vi "WriteToTarget_20190401.vi"(8 "error in":errorcluster, 11 "Tones":T1={"Config"={"UsrCfg"={"Paths"={"CfgFile"=path "", "LogFolder"=path "", "LogFile"=path "", "NAS path"=path "", "ThreshFile"=path "", "RedunFolder"=path ""}, "SampleRate"=0.0}, "FP_User"={"#NoiseSums"=1, "Max_df"=1, "AvgAvg"=FALSE, "#Avg"=0, "AutoCenter"=FALSE, "Inclin"={"Vmin"=0.0, "Vmax"=0.0, "Angle_min"=0.0, "Angle_max"=0.0, "Offset"=0.0, "Pos_Neg"=FALSE}, "1"={"Cal_"={"Fine"=0.0, "Coarse_"=0.0}, "Beac"={"Fine"=0.0, "Coarse_"=0.0}, "Scale"={"Step4"=0.0, "Step5"=0.0, "Step6"=0.0, "Step7"=0.0}, "Offset"=0.0, "Scale_Noise"=0.0, "Scale_Step1"=0.0, "Scale_In_RT"=0.0, "ScaleMeas"=0.0, "FreqsToRemove"=[], "Width"=[0, 1633], "ScaleMeasEnum"=enum."50", "FilterEnab"=enum."Step 1"}, "2"={"Cal_"={"Fine"=0.0, "Coarse_"=0.0}, "Beac"={"Fine"=0.0, "Coarse_"=0.0}, "Scale"={"Step4"=0.0, "Step5"=0.0, "Step6"=0.0, "Step7"=0.0}, "Offset"=0.0, "Scale_Noise"=0.0, "Scale_Step1"=0.0, "Scale_In_RT"=0.0, "ScaleMeas"=0.0, "FreqsToRemove"=[], "Width"=[0, 1633], "ScaleMeasEnum"=enum."50", "FilterEnab"=enum."Step 1"}, "3"={"Cal_"={"Fine"=0.0, "Coarse_"=0.0}, "Beac"={"Fine"=0.0, "Coarse_"=0.0}, "Scale"={"Step4"=0.0, "Step5"=0.0, "Step6"=0.0, "Step7"=0.0}, "Offset"=0.0, "Scale_Noise"=0.0, "Scale_Step1"=0.0, "Scale_In_RT"=0.0, "ScaleMeas"=0.0, "FreqsToRemove"=[], "Width"=[0, 1633], "ScaleMeasEnum"=enum."50", "FilterEnab"=enum."Step 1"}, "4"={"Cal_"={"Fine"=0.0, "Coarse_"=0.0}, "Beac"={"Fine"=0.0, "Coarse_"=0.0}, "Scale"={"Step4"=0.0, "Step5"=0.0, "Step6"=0.0, "Step7"=0.0}, "Offset"=0.0, "Scale_Noise"=0.0, "Scale_Step1"=0.0, "Scale_In_RT"=0.0, "ScaleMeas"=0.0, "FreqsToRemove"=[], "Width"=[0, 1633], "ScaleMeasEnum"=enum."50", "FilterEnab"=enum."Step 1"}, "Target to Probe"=enum."4", "SNR_Thresh"=1.0, "Paths"={"CfgFile"=path "", "LogFolder"=path "", "LogFile"=path "", "NAS path"=path "", "ThreshFile"=path "", "RedunFolder"=path ""}, "Connex_Location"="", "SimulateFPGA"=FALSE, "Deadband"=0.0}}, "FPGA"={"Target"=enum."4", "Channel"=enum."4", "Ref1"=refnum, "Ref2"=refnum}, "Now"={"Target"=enum."1", "SampleRate"=0.0, "AvgFreq"=0.0, "72_Shift_"=-24999462.633451957, "84_Shift_"=-24999462.633451957, "1"={"Cal"={"Shift_"=0.0, "Peak_ToFPGA"=-24999462.633451957, "MaxValue"=0.0, "MaxIndex"=0, "Tone"={"PkLocTrak"=0.0, "PkLocDisp"=0.0, "df_"=0.0, "ZoomPwr"=[], "Phase"=0.0, "PhaseOld"=0.0, "AboveThresh?"=FALSE, "MaxI"=0.0, "MaxQ"=0.0, "median"=0.0, "ISpect"=[], "QSpect"=[], "DeltaPhase"=0.0}, "TimeDomainI"=[], "TimeDomainQ"=array[12500 elements], "PwrSpectrum"=[], "RunningAvgFreq"=0.0, "ISpectPos"=[], "ISpectNeg"=[], "QSpectPos"=[], "QSpectNeg"=[], "10Hz_PwrSpectr"=[], "SNR"=0.0, "AliasWarn"=FALSE, "10Hz_Peak"=[], "ISpect+-"=[], "QSpect+-"=[], "TimeStamp"=timestamp(0 s since 1904-01-01), "I_Index"=array[12500 elements], "Q_Index"=array[12500 elements], "10MHz"=FALSE}, "Beac"={"Shift_"=0.0, "Peak_ToFPGA"=-24999462.633451957, "MaxValue"=0.0, "MaxIndex"=0, "Tone"={"PkLocTrak"=0.0, "PkLocDisp"=0.0, "df_"=0.0, "ZoomPwr"=[], "Phase"=0.0, "PhaseOld"=0.0, "AboveThresh?"=FALSE, "MaxI"=0.0, "MaxQ"=0.0, "median"=0.0, "ISpect"=[], "QSpect"=[], "DeltaPhase"=0.0}, "TimeDomainI"=[], "TimeDomainQ"=array[12500 elements], "PwrSpectrum"=[], "RunningAvgFreq"=0.0, "ISpectPos"=[], "ISpectNeg"=[], "QSpectPos"=[], "QSpectNeg"=[], "10Hz_PwrSpectr"=[], "SNR"=0.0, "AliasWarn"=FALSE, "10Hz_Peak"=[], "ISpect+-"=[], "QSpect+-"=[], "TimeStamp"=timestamp(0 s since 1904-01-01), "I_Index"=array[12500 elements], "Q_Index"=array[12500 elements], "10MHz"=FALSE}, "Time"=[], "Saturat"={"MeasMean0"=0.0, "MeasMean1"=0.0, "MeasMax"=0.0, "1_Max"=0.0, "4_Max"=0.0, "5_Max"=0.0, "6_Max"=0.0, "7_Max"=0.0}}, "2"={"Cal"={"Shift_"=0.0, "Peak_ToFPGA"=-24999462.633451957, "MaxValue"=0.0, "MaxIndex"=0, "Tone"={"PkLocTrak"=0.0, "PkLocDisp"=0.0, "df_"=0.0, "ZoomPwr"=[], "Phase"=0.0, "PhaseOld"=0.0, "AboveThresh?"=FALSE, "MaxI"=0.0, "MaxQ"=0.0, "median"=0.0, "ISpect"=[], "QSpect"=[], "DeltaPhase"=0.0}, "TimeDomainI"=[], "TimeDomainQ"=array[12500 elements], "PwrSpectrum"=[], "RunningAvgFreq"=0.0, "ISpectPos"=[], "ISpectNeg"=[], "QSpectPos"=[], "QSpectNeg"=[], "10Hz_PwrSpectr"=[], "SNR"=0.0, "AliasWarn"=FALSE, "10Hz_Peak"=[], "ISpect+-"=[], "QSpect+-"=[], "TimeStamp"=timestamp(0 s since 1904-01-01), "I_Index"=array[12500 elements], "Q_Index"=array[12500 elements], "10MHz"=FALSE}, "Beac"={"Shift_"=0.0, "Peak_ToFPGA"=-24999462.633451957, "MaxValue"=0.0, "MaxIndex"=0, "Tone"={"PkLocTrak"=0.0, "PkLocDisp"=0.0, "df_"=0.0, "ZoomPwr"=[], "Phase"=0.0, "PhaseOld"=0.0, "AboveThresh?"=FALSE, "MaxI"=0.0, "MaxQ"=0.0, "median"=0.0, "ISpect"=[], "QSpect"=[], "DeltaPhase"=0.0}, "TimeDomainI"=[], "TimeDomainQ"=array[12500 elements], "PwrSpectrum"=[], "RunningAvgFreq"=0.0, "ISpectPos"=[], "ISpectNeg"=[], "QSpectPos"=[], "QSpectNeg"=[], "10Hz_PwrSpectr"=[], "SNR"=0.0, "AliasWarn"=FALSE, "10Hz_Peak"=[], "ISpect+-"=[], "QSpect+-"=[], "TimeStamp"=timestamp(0 s since 1904-01-01), "I_Index"=array[12500 elements], "Q_Index"=array[12500 elements], "10MHz"=FALSE}, "Time"=[], "Saturat"={"MeasMean0"=0.0, "MeasMean1"=0.0, "MeasMax"=0.0, "1_Max"=0.0, "4_Max"=0.0, "5_Max"=0.0, "6_Max"=0.0, "7_Max"=0.0}}, "3"={"Cal"={"Shift_"=0.0, "Peak_ToFPGA"=-24999462.633451957, "MaxValue"=0.0, "MaxIndex"=0, "Tone"={"PkLocTrak"=0.0, "PkLocDisp"=0.0, "df_"=0.0, "ZoomPwr"=[], "Phase"=0.0, "PhaseOld"=0.0, "AboveThresh?"=FALSE, "MaxI"=0.0, "MaxQ"=0.0, "median"=0.0, "ISpect"=[], "QSpect"=[], "DeltaPhase"=0.0}, "TimeDomainI"=[], "TimeDomainQ"=array[12500 elements], "PwrSpectrum"=[], "RunningAvgFreq"=0.0, "ISpectPos"=[], "ISpectNeg"=[], "QSpectPos"=[], "QSpectNeg"=[], "10Hz_PwrSpectr"=[], "SNR"=0.0, "AliasWarn"=FALSE, "10Hz_Peak"=[], "ISpect+-"=[], "QSpect+-"=[], "TimeStamp"=timestamp(0 s since 1904-01-01), "I_Index"=array[12500 elements], "Q_Index"=array[12500 elements], "10MHz"=FALSE}, "Beac"={"Shift_"=0.0, "Peak_ToFPGA"=-24999462.633451957, "MaxValue"=0.0, "MaxIndex"=0, "Tone"={"PkLocTrak"=0.0, "PkLocDisp"=0.0, "df_"=0.0, "ZoomPwr"=[], "Phase"=0.0, "PhaseOld"=0.0, "AboveThresh?"=FALSE, "MaxI"=0.0, "MaxQ"=0.0, "median"=0.0, "ISpect"=[], "QSpect"=[], "DeltaPhase"=0.0}, "TimeDomainI"=[], "TimeDomainQ"=array[12500 elements], "PwrSpectrum"=[], "RunningAvgFreq"=0.0, "ISpectPos"=[], "ISpectNeg"=[], "QSpectPos"=[], "QSpectNeg"=[], "10Hz_PwrSpectr"=[], "SNR"=0.0, "AliasWarn"=FALSE, "10Hz_Peak"=[], "ISpect+-"=[], "QSpect+-"=[], "TimeStamp"=timestamp(0 s since 1904-01-01), "I_Index"=array[12500 elements], "Q_Index"=array[12500 elements], "10MHz"=FALSE}, "Time"=[], "Saturat"={"MeasMean0"=0.0, "MeasMean1"=0.0, "MeasMax"=0.0, "1_Max"=0.0, "4_Max"=0.0, "5_Max"=0.0, "6_Max"=0.0, "7_Max"=0.0}}, "4"={"Cal"={"Shift_"=0.0, "Peak_ToFPGA"=-24999462.633451957, "MaxValue"=0.0, "MaxIndex"=0, "Tone"={"PkLocTrak"=0.0, "PkLocDisp"=0.0, "df_"=0.0, "ZoomPwr"=[], "Phase"=0.0, "PhaseOld"=0.0, "AboveThresh?"=FALSE, "MaxI"=0.0, "MaxQ"=0.0, "median"=0.0, "ISpect"=[], "QSpect"=[], "DeltaPhase"=0.0}, "TimeDomainI"=[], "TimeDomainQ"=array[12500 elements], "PwrSpectrum"=[], "RunningAvgFreq"=0.0, "ISpectPos"=[], "ISpectNeg"=[], "QSpectPos"=[], "QSpectNeg"=[], "10Hz_PwrSpectr"=[], "SNR"=0.0, "AliasWarn"=FALSE, "10Hz_Peak"=[], "ISpect+-"=[], "QSpect+-"=[], "TimeStamp"=timestamp(0 s since 1904-01-01), "I_Index"=array[12500 elements], "Q_Index"=array[12500 elements], "10MHz"=FALSE}, "Beac"={"Shift_"=0.0, "Peak_ToFPGA"=-24999462.633451957, "MaxValue"=0.0, "MaxIndex"=0, "Tone"={"PkLocTrak"=0.0, "PkLocDisp"=0.0, "df_"=0.0, "ZoomPwr"=[], "Phase"=0.0, "PhaseOld"=0.0, "AboveThresh?"=FALSE, "MaxI"=0.0, "MaxQ"=0.0, "median"=0.0, "ISpect"=[], "QSpect"=[], "DeltaPhase"=0.0}, "TimeDomainI"=[], "TimeDomainQ"=array[12500 elements], "PwrSpectrum"=[], "RunningAvgFreq"=0.0, "ISpectPos"=[], "ISpectNeg"=[], "QSpectPos"=[], "QSpectNeg"=[], "10Hz_PwrSpectr"=[], "SNR"=0.0, "AliasWarn"=FALSE, "10Hz_Peak"=[], "ISpect+-"=[], "QSpect+-"=[], "TimeStamp"=timestamp(0 s since 1904-01-01), "I_Index"=array[12500 elements], "Q_Index"=array[12500 elements], "10MHz"=FALSE}, "Time"=[], "Saturat"={"MeasMean0"=0.0, "MeasMean1"=0.0, "MeasMax"=0.0, "1_Max"=0.0, "4_Max"=0.0, "5_Max"=0.0, "6_Max"=0.0, "7_Max"=0.0}}}, "FreqFiles"={"72"=path "", "84"=path ""}} {"Now"."4"."Beac"."Tone"."median" format="%0.2f"; "Now"."4"."Beac"."Tone"."MaxQ" format="%0.2f"; "Now"."4"."Cal"."Tone"."median" format="%0.2f"; "Now"."4"."Cal"."Tone"."MaxQ" format="%0.2f"; "Now"."3"."Beac"."Tone"."median" format="%0.2f"; "Now"."3"."Beac"."Tone"."MaxQ" format="%0.2f"; "Now"."3"."Cal"."Tone"."median" format="%0.2f"; "Now"."3"."Cal"."Tone"."MaxQ" format="%0.2f"; "Now"."2"."Beac"."Tone"."median" format="%0.2f"; "Now"."2"."Beac"."Tone"."MaxQ" format="%0.2f"; "Now"."2"."Cal"."Tone"."median" format="%0.2f"; "Now"."2"."Cal"."Tone"."MaxQ" format="%0.2f"; "Now"."1"."Beac"."Tone"."median" format="%0.2f"; "Now"."1"."Beac"."Tone"."MaxQ" format="%0.2f"; "Now"."1"."Cal"."Tone"."median" format="%0.2f"; "Now"."1"."Cal"."Tone"."MaxQ" format="%0.2f"; "Config"."FP_User"."Deadband" format="%#.0f"}) -> (0 "error out":errorcluster)   [LabVIEW 2018]
uses:
  Controls/Clusts/Tones_Loop.ctl
  Controls/Clusts/Config_Clust.ctl
  Controls/Clusts/UserConfig.ctl
  Controls/PathsCluster.ctl
  Controls/Clusts/FrontPanel_UserConfig.ctl
  Controls/Clusts/Inclinometer_User_Cfg.ctl
  Controls/Clusts/FP_UserTargetConfig.ctl
  Controls/Clusts/FreqShift.ctl
  Controls/Clusts/FPGA_Scale.ctl
  Controls/Enums/ScaleMeasure.ctl
  Controls/RadioButtons/FilterEnableRadio.ctl
  Controls/Enums/TargetNumber.ctl
  Controls/Clusts/FPGA_Config_Clust.ctl
  Controls/Clusts/NowAllTones.ctl
  Controls/Clusts/TargetToneData.ctl
  Controls/Clusts/ChannelToneData.ctl
  Controls/ToneInfoClust.ctl
  Controls/Clusts/SaturationMonitor.ctl
  Controls/Clusts/FreqFilePaths.ctl
  <vilib>/Utility/error.llb/Error Cluster From Error Code.vi
  <vilib>/rvi/errors/niLvFpgaAdjustHostInterfaceError.vi
  <vilib>/rvi/interface/nirviReadWriteControl/nirviReadWriteControl.xnode
  NiFpgaLv.dll
  <vilib>/rvi/interface/Simulation/niFpgaSimulationCallBeginRW.vi
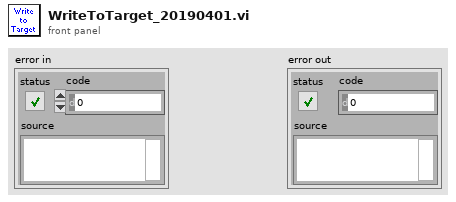
[diagram p1: front panel]
types:
  T1 = typedef "Tones_Loop.ctl" = cluster{"Config":T2, "FPGA":T13, "Now":T14, "FreqFiles":T19}
  T2 = typedef "Config_Clust.ctl" = cluster{"UsrCfg":T3, "FP_User":T5}
  T3 = typedef "UserConfig.ctl" = cluster{"Paths":T4, "SampleRate":dbl}
  T4 = typedef "PathsCluster.ctl" = cluster{"CfgFile":path, "LogFolder":path, "LogFile":path, "NAS path":path, "ThreshFile":path, "RedunFolder":path}
  T5 = typedef "FrontPanel_UserConfig.ctl" = cluster{"#NoiseSums":u32, "Max_df":u32, "AvgAvg":bool, "#Avg":u16, "AutoCenter":bool, "Inclin":T6, "1":T7, "2":T7, "3":T7, "4":T7, "Target to Probe":T12, "SNR_Thresh":dbl, "Paths":T4, "Connex_Location":string, "SimulateFPGA":bool, "Deadband":dbl}
  T6 = typedef "Inclinometer_User_Cfg.ctl" = cluster{"Vmin":dbl, "Vmax":dbl, "Angle_min":dbl, "Angle_max":dbl, "Offset":dbl, "Pos_Neg":bool}
  T7 = typedef "FP_UserTargetConfig.ctl" = cluster{"Cal_":T8, "Beac":T8, "Scale":T9, "Offset":fxp<+/-,16,16>, "Scale_Noise":fxp<+/-,30,30>, "Scale_Step1":fxp<+/-,17,17>, "Scale_In_RT":ext, "ScaleMeas":fxp<+/-,16,1>, "FreqsToRemove":i32[], "Width":i32[], "ScaleMeasEnum":T10, "FilterEnab":T11}
  T8 = typedef "FreqShift.ctl" = cluster{"Fine":dbl, "Coarse_":dbl}
  T9 = typedef "FPGA_Scale.ctl" = cluster{"Step4":fxp<+/-,23,23>, "Step5":fxp<+/-,23,23>, "Step6":fxp<+/-,23,23>, "Step7":fxp<+/-,23,23>}
  T10 = typedef "ScaleMeasure.ctl" = enum16{"1", "10", "50", "42"}
  T11 = typedef "FilterEnableRadio.ctl" = enum32{"None", "Step 1", "Frequency Shift", "Step 4", "Step 5", "Step 6", "Step 7"}
  T12 = typedef "TargetNumber.ctl" = enum16{"1", "2", "3", "4"}
  T13 = typedef "FPGA_Config_Clust.ctl" = cluster{"Target":T12, "Channel":T12, "Ref1":refnum<k20>, "Ref2":refnum<k20>}
  T14 = typedef "NowAllTones.ctl" = cluster{"Target":T12, "SampleRate":dbl, "AvgFreq":dbl, "72_Shift_":dbl, "84_Shift_":dbl, "1":T15, "2":T15, "3":T15, "4":T15}
  T15 = typedef "TargetToneData.ctl" = cluster{"Cal":T16, "Beac":T16, "Time":timestamp[], "Saturat":T18}
  T16 = typedef "ChannelToneData.ctl" = cluster{"Shift_":dbl, "Peak_ToFPGA":dbl, "MaxValue":dbl, "MaxIndex":i32, "Tone":T17, "TimeDomainI":ext[], "TimeDomainQ":ext[], "PwrSpectrum":dbl[], "RunningAvgFreq":dbl, "ISpectPos":dbl[], "ISpectNeg":dbl[], "QSpectPos":dbl[], "QSpectNeg":dbl[], "10Hz_PwrSpectr":dbl[][], "SNR":dbl, "AliasWarn":bool, "10Hz_Peak":dbl[], "ISpect+-":dbl[], "QSpect+-":dbl[], "TimeStamp":timestamp, "I_Index":ext[], "Q_Index":ext[], "10MHz":bool}
  T17 = typedef "ToneInfoClust.ctl" = cluster{"PkLocTrak":dbl, "PkLocDisp":dbl, "df_":dbl, "ZoomPwr":dbl[], "Phase":dbl, "PhaseOld":dbl, "AboveThresh?":bool, "MaxI":dbl, "MaxQ":dbl, "median":dbl, "ISpect":dbl[], "QSpect":dbl[], "DeltaPhase":dbl}
  T18 = typedef "SaturationMonitor.ctl" = cluster{"MeasMean0":dbl, "MeasMean1":dbl, "MeasMax":dbl, "1_Max":dbl, "4_Max":dbl, "5_Max":dbl, "6_Max":dbl, "7_Max":dbl}
  T19 = typedef "FreqFilePaths.ctl" = cluster{"72":path, "84":path}
  T20 = typedef "FPGA_Filter_Enable.ctl" = cluster{"FreqShiftEnable":bool, "Step4Enable":bool, "Step5Enable":bool, "Step6Enable":bool, "Step7Enable":bool}
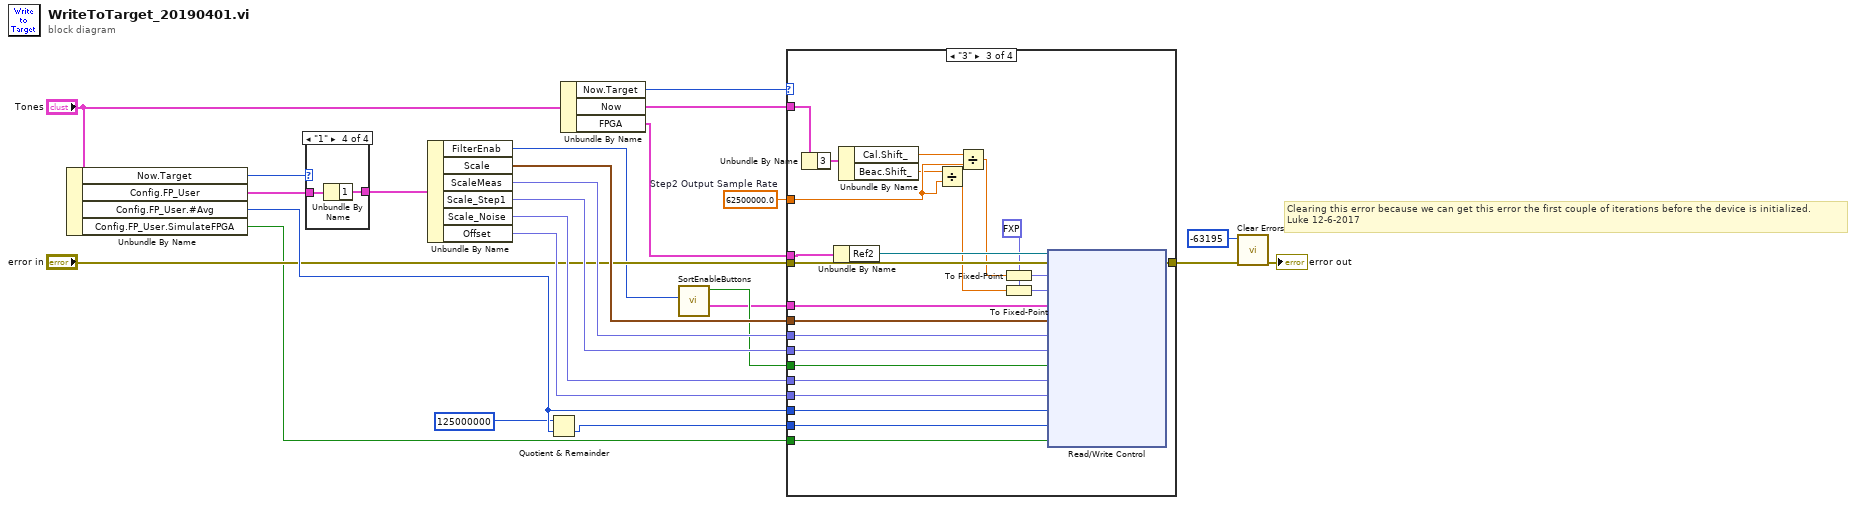
[diagram p0: block diagram]
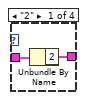
[diagram p2: hidden frame]
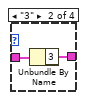
[diagram p3: hidden frame]
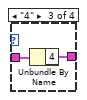
[diagram p4: hidden frame]
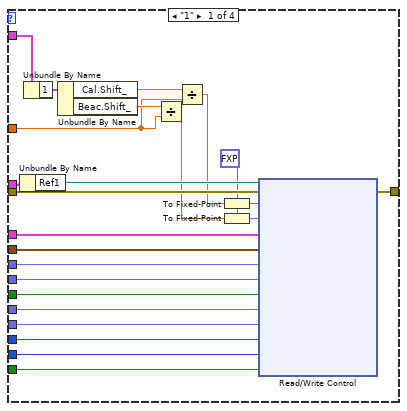
[diagram p5: hidden frame]
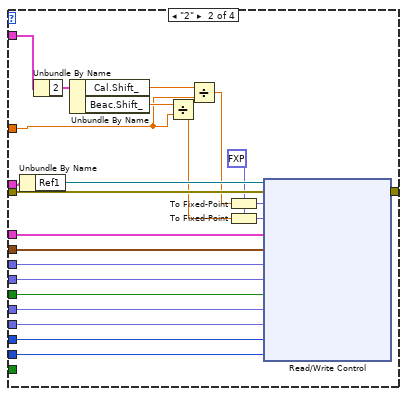
[diagram p6: hidden frame]
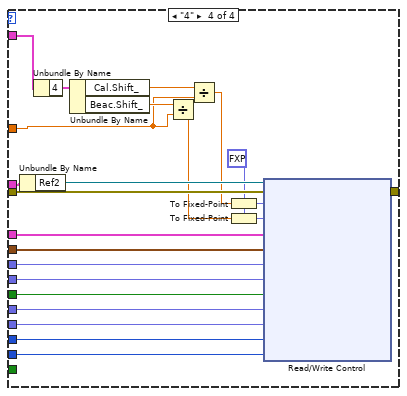
[diagram p7: hidden frame]
diagram:
  w7 = 62500000.0  # Step2 Output Sample Rate
  # "Clearing this error because we can get this error the first couple of iterations before the device is initialized.\nLuke 12-6-2017"
  n1 = Unbundle By Name("Tones") -> ("Now.Target"=w22:T12, "Config.FP_User"=w18:T5, "Config.FP_User.#Avg"=w20:u16, "Config.FP_User.SimulateFPGA"=w1:bool)
  n2 = case shown="\"1\"" w22 {
    tunnel: w18 -> [w26 w28 w30 w32]
    tunnel: [w25 w27 w29 w31] -> w19
    frame "2" {
      n3 = Unbundle By Name(w26) -> ("2"=w25:T7)
    }
    frame "3" {
      n4 = Unbundle By Name(w28) -> ("3"=w27:T7)
    }
    frame "4" {
      n5 = Unbundle By Name(w30) -> ("4"=w29:T7)
    }
    frame "1" {
      n6 = Unbundle By Name(w32) -> ("1"=w31:T7)
    }
  }
  n7 = Unbundle By Name(w19) -> ("FilterEnab"=w4:T11, "Scale"=w12:T9, "ScaleMeas"=w13:fxp<+/-,16,1>, "Scale_Step1"=w14:fxp<+/-,17,17>, "Scale_Noise"=w15:fxp<+/-,30,30>, "Offset"=w16:fxp<+/-,16,16>)
  n8 = Quotient & Remainder(x=u32 125000000, y=w20) -> (floor(x/y)=w10:u32)  [unwired: 1 out]
  n9 = Unbundle By Name("Tones") -> ("Now.Target"=w24:T12, "Now"=w8:T14, "FPGA"=w23:T13)
  n10 = call "SortEnableButtons.vi"("Radio Buttons"=w4) -> ("Enable out"=w2:T20, "EnableStep1 out"=w3:bool)  [unwired: 8 in, 1 out]
  n11 = case shown="\"3\"" w24 {
    tunnel: w10 -> [w56 w79 w103 w126]
    tunnel: "error in" -> [w55 w78 w102 w125]
    tunnel: w2 -> [w54 w77 w101 w124]
    tunnel: w12 -> [w53 w76 w100 w123]
    tunnel: w13 -> [w52 w75 w99 w122]
    tunnel: w14 -> [w51 w74 w98 w121]
    tunnel: w3 -> [w50 w73 w97 w120]
    tunnel: w15 -> [w49 w72 w96 w119]
    tunnel: w16 -> [w48 w71 w95 w118]
    tunnel: [w47 w70 w94 w117] -> w17
    tunnel: w20 -> [w46 w69 w93 w116]
    tunnel: w23 -> [w45 w68 w92 w115]
    tunnel: w8 -> [w43 w63 w91 w110]
    tunnel: w7 -> [w39 w62 w89 w109]
    tunnel: w1 -> [w33 _ w80 _]
    frame "1" {
      w36 = fxp<+/-,48,0> 0.0 ("FreqShiftCal")
      n12 = Unbundle By Name(w45) -> ("Ref1"=w44:refnum<k20>)
      n13 = Unbundle By Name(w43) -> ("1"=w42:T15)
      n14 = Unbundle By Name(w42) -> ("Cal.Shift_"=w41:dbl, "Beac.Shift_"=w40:dbl)
      n15 = Divide(x=w40, y=w39) -> (x/y=w34:dbl)
      n16 = Divide(x=w41, y=w39) -> (x/y=w35:dbl)
      n17 = To Fixed-Point(fixed-point type=w36, number=w35) -> (fixed-point=w38:fxp<+/-,48,0>)
      n18 = To Fixed-Point(fixed-point type=w36, number=w34) -> (fixed-point=w37:fxp<+/-,48,0>)
      n19 = xnode "Read/Write Control"("FPGA VI Reference In"=w44, "error in"=w55, "FreqShiftCal"=w38, "FreqShiftBeac"=w37, "Enable"=w54, "Scale"=w53, "ScaleMeasurement"=w52, "Scale_Step1"=w51, "EnableStep1"=w50, "Scale_NoiseFloor"=w49, "Offset"=w48, "#Avg"=w46, "SampleCountReset"=w56, "Simulate?"=w33) -> ("error out"=w47:errorcluster)  [unwired: 1 out]
    }
    frame "2" {
      w61 = fxp<+/-,48,0> 0.0 ("FreqShiftCal")
      n20 = Unbundle By Name(w68) -> ("Ref1"=w67:refnum<k20>)
      n21 = Unbundle By Name(w63) -> ("2"=w66:T15)
      n22 = Unbundle By Name(w66) -> ("Cal.Shift_"=w65:dbl, "Beac.Shift_"=w64:dbl)
      n23 = Divide(x=w64, y=w62) -> (x/y=w57:dbl)
      n24 = Divide(x=w65, y=w62) -> (x/y=w60:dbl)
      n25 = To Fixed-Point(fixed-point type=w61, number=w60) -> (fixed-point=w59:fxp<+/-,48,0>)
      n26 = To Fixed-Point(fixed-point type=w61, number=w57) -> (fixed-point=w58:fxp<+/-,48,0>)
      n27 = xnode "Read/Write Control"("FPGA VI Reference In"=w67, "error in"=w78, "FreqShiftCal 2"=w59, "FreqShiftBeac 2"=w58, "Enable 2"=w77, "Scale 2"=w76, "ScaleMeasurement 2"=w75, "Scale_Step1_2"=w74, "EnableStep1_2"=w73, "Scale_NoiseFloor 2"=w72, "Offset 2"=w71, "#Avg 2"=w69, "SampleCountReset 2"=w79) -> ("error out"=w70:errorcluster)  [unwired: 1 out]
    }
    frame "3" {
      w85 = fxp<+/-,48,0> 0.0 ("FreqShiftCal")
      n28 = Unbundle By Name(w91) -> ("3"=w90:T15)
      n29 = Unbundle By Name(w92) -> ("Ref2"=w88:refnum<k20>)
      n30 = Unbundle By Name(w90) -> ("Cal.Shift_"=w87:dbl, "Beac.Shift_"=w86:dbl)
      n31 = Divide(x=w86, y=w89) -> (x/y=w82:dbl)
      n32 = Divide(x=w87, y=w89) -> (x/y=w81:dbl)
      n33 = To Fixed-Point(fixed-point type=w85, number=w81) -> (fixed-point=w84:fxp<+/-,48,0>)
      n34 = To Fixed-Point(fixed-point type=w85, number=w82) -> (fixed-point=w83:fxp<+/-,48,0>)
      n35 = xnode "Read/Write Control"("FPGA VI Reference In"=w88, "error in"=w102, "FreqShiftCal"=w84, "FreqShiftBeac"=w83, "Enable"=w101, "Scale"=w100, "ScaleMeasurement"=w99, "Scale_Step1"=w98, "EnableStep1"=w97, "Scale_NoiseFloor"=w96, "Offset"=w95, "#Avg"=w93, "SampleCountReset"=w103, "Simulate?"=w80) -> ("error out"=w94:errorcluster)  [unwired: 1 out]
    }
    frame "4" {
      w108 = fxp<+/-,48,0> 0.0 ("FreqShiftCal")
      n36 = Unbundle By Name(w115) -> ("Ref2"=w114:refnum<k20>)
      n37 = Unbundle By Name(w110) -> ("4"=w113:T15)
      n38 = Unbundle By Name(w113) -> ("Cal.Shift_"=w112:dbl, "Beac.Shift_"=w111:dbl)
      n39 = Divide(x=w111, y=w109) -> (x/y=w104:dbl)
      n40 = Divide(x=w112, y=w109) -> (x/y=w107:dbl)
      n41 = To Fixed-Point(fixed-point type=w108, number=w107) -> (fixed-point=w106:fxp<+/-,48,0>)
      n42 = To Fixed-Point(fixed-point type=w108, number=w104) -> (fixed-point=w105:fxp<+/-,48,0>)
      n43 = xnode "Read/Write Control"("FPGA VI Reference In"=w114, "error in"=w125, "FreqShiftCal 2"=w106, "FreqShiftBeac 2"=w105, "Enable 2"=w124, "Scale 2"=w123, "ScaleMeasurement 2"=w122, "Scale_Step1_2"=w121, "EnableStep1_2"=w120, "Scale_NoiseFloor 2"=w119, "Offset 2"=w118, "#Avg 2"=w116, "SampleCountReset 2"=w126) -> ("error out"=w117:errorcluster)  [unwired: 1 out]
    }
  }
  n44 = call <vilib>:"Clear Errors.vi"("error in (no error)"=w17, "specific error code to clear (0: all)"=-63195) -> ("error out"=→"error out":errorcluster)  [unwired: 4 in, 1 out]
